vi "test Parse DBL Array3.vi"(11 "Test Case In":refnum<class "Test Simple CSV Parser.lvclass">) -> (0 "error out":errorcluster, 3 "Test Case Out":refnum<class "Test Simple CSV Parser.lvclass">)   [LabVIEW 2024, in "Test Simple CSV Parser.lvclass"]
uses:
  Test Simple CSV Parser.lvclass
  Test Simple CSV Parser.lvclass/Test Simple CSV Parser.ctl
  CSV Parser/Simple CSV Parser/Simple CSV Parser.lvclass
  <vilib>/Astemes/LUnit/Test Case.lvclass
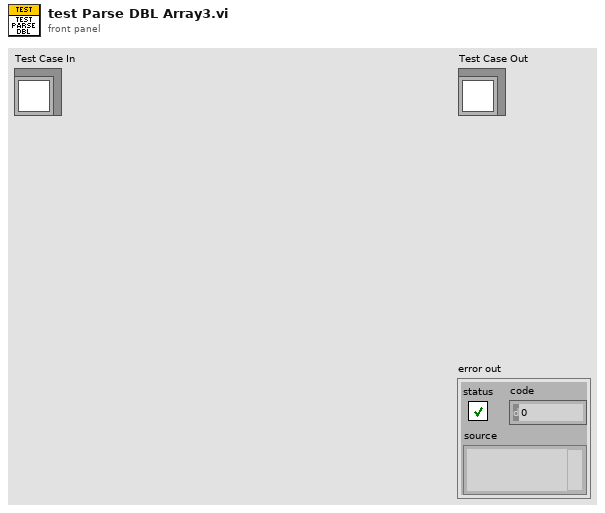
[diagram p1: front panel]
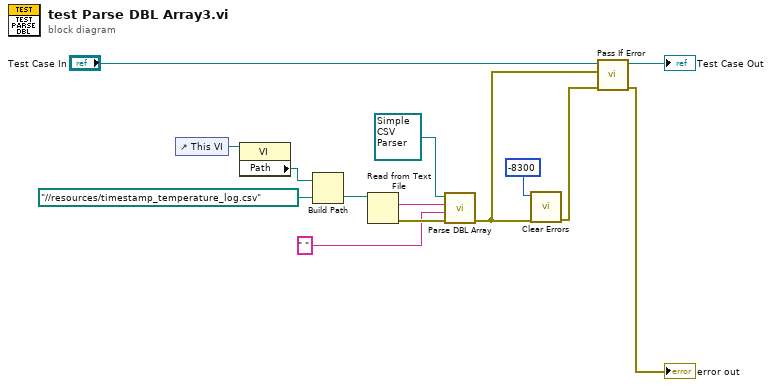
[diagram p0: block diagram]
diagram:
  n1 = control-ref of="This VI"() -> (w5:refnum<vi>)
  n2 = property class="VI"(reference=w5) -> ("Path"=w4:path)  [unwired: 1 in, 2 out]
  n3 = Build Path(base path=w4, name or relative path=path "../../resources/timestamp_temperature_log.csv" ("file (use dialog)")) -> (appended path=w7:path)
  n4 = Read from Text File(file (use dialog)=w7) -> (text=w2:string, error out=w3:errorcluster)  [unwired: 3 in, 2 out]
  n5 = call-dynamic "Parse DBL Array.vi"("error in"=w3, "Input <JSON>"=" ", "csv string"=w2, "Simple CSV Parser in"=refnum<class "Simple CSV Parser.lvclass"> refnum) -> ("error out"=w9:errorcluster)  [unwired: 5 in, 2 out]
  n6 = call <vilib>:"Clear Errors.vi"("error in (no error)"=w9, "specific error code to clear (0: all)"=-8300) -> ("error out"=w8:errorcluster)  [unwired: 4 in, 1 out]
  n7 = call <vilib>:"Pass If Error.vi"("error in (no error)"=w8, "Assert error"=w9, "LUnit Test Case In"="Test Case In") -> ("error out"=→"error out":errorcluster, "LUnit Test Case Out"=→"Test Case Out":refnum<class "Test Simple CSV Parser.lvclass">)  [unwired: 7 in]
